vi "VISJS Viewer.vi"(4 "Extra Scripts":string, 5 "FileDependency out":map{path, T1}(c390), 6 "Options":string, 7 "OpenWebBrowser(False)":bool, 8 "error in":errorcluster, 9 "Embedd VISJS Librarya in HTMl File(False)":bool, 10 "HTMLFilePath":path, 11 "LibraryDependency":map{path, T3}(c390)) -> (0 "error out":errorcluster, 3 "HTMLFileContent":string)   [LabVIEW 2020, in "VISJS Viewer.lvlib"]
uses:
  VISJS Viewer.lvlib
  DependencyChecker/LibraryDependentInfo.vi
  <vilib>/Utility/lvfile.llb/FT_FileTypes.ctl
  DependencyChecker/FileDependencyType.ctl
  <vilib>/Utility/miscctls.llb/LVMapReplaceAction.ctl
  <vilib>/Platform/browser.llb/Open URL in Default Browser (path).vi
  <vilib>/Utility/lvfile.llb/NI_FileType.lvlib
  DependencyChecker/DependencyChecker.lvlib
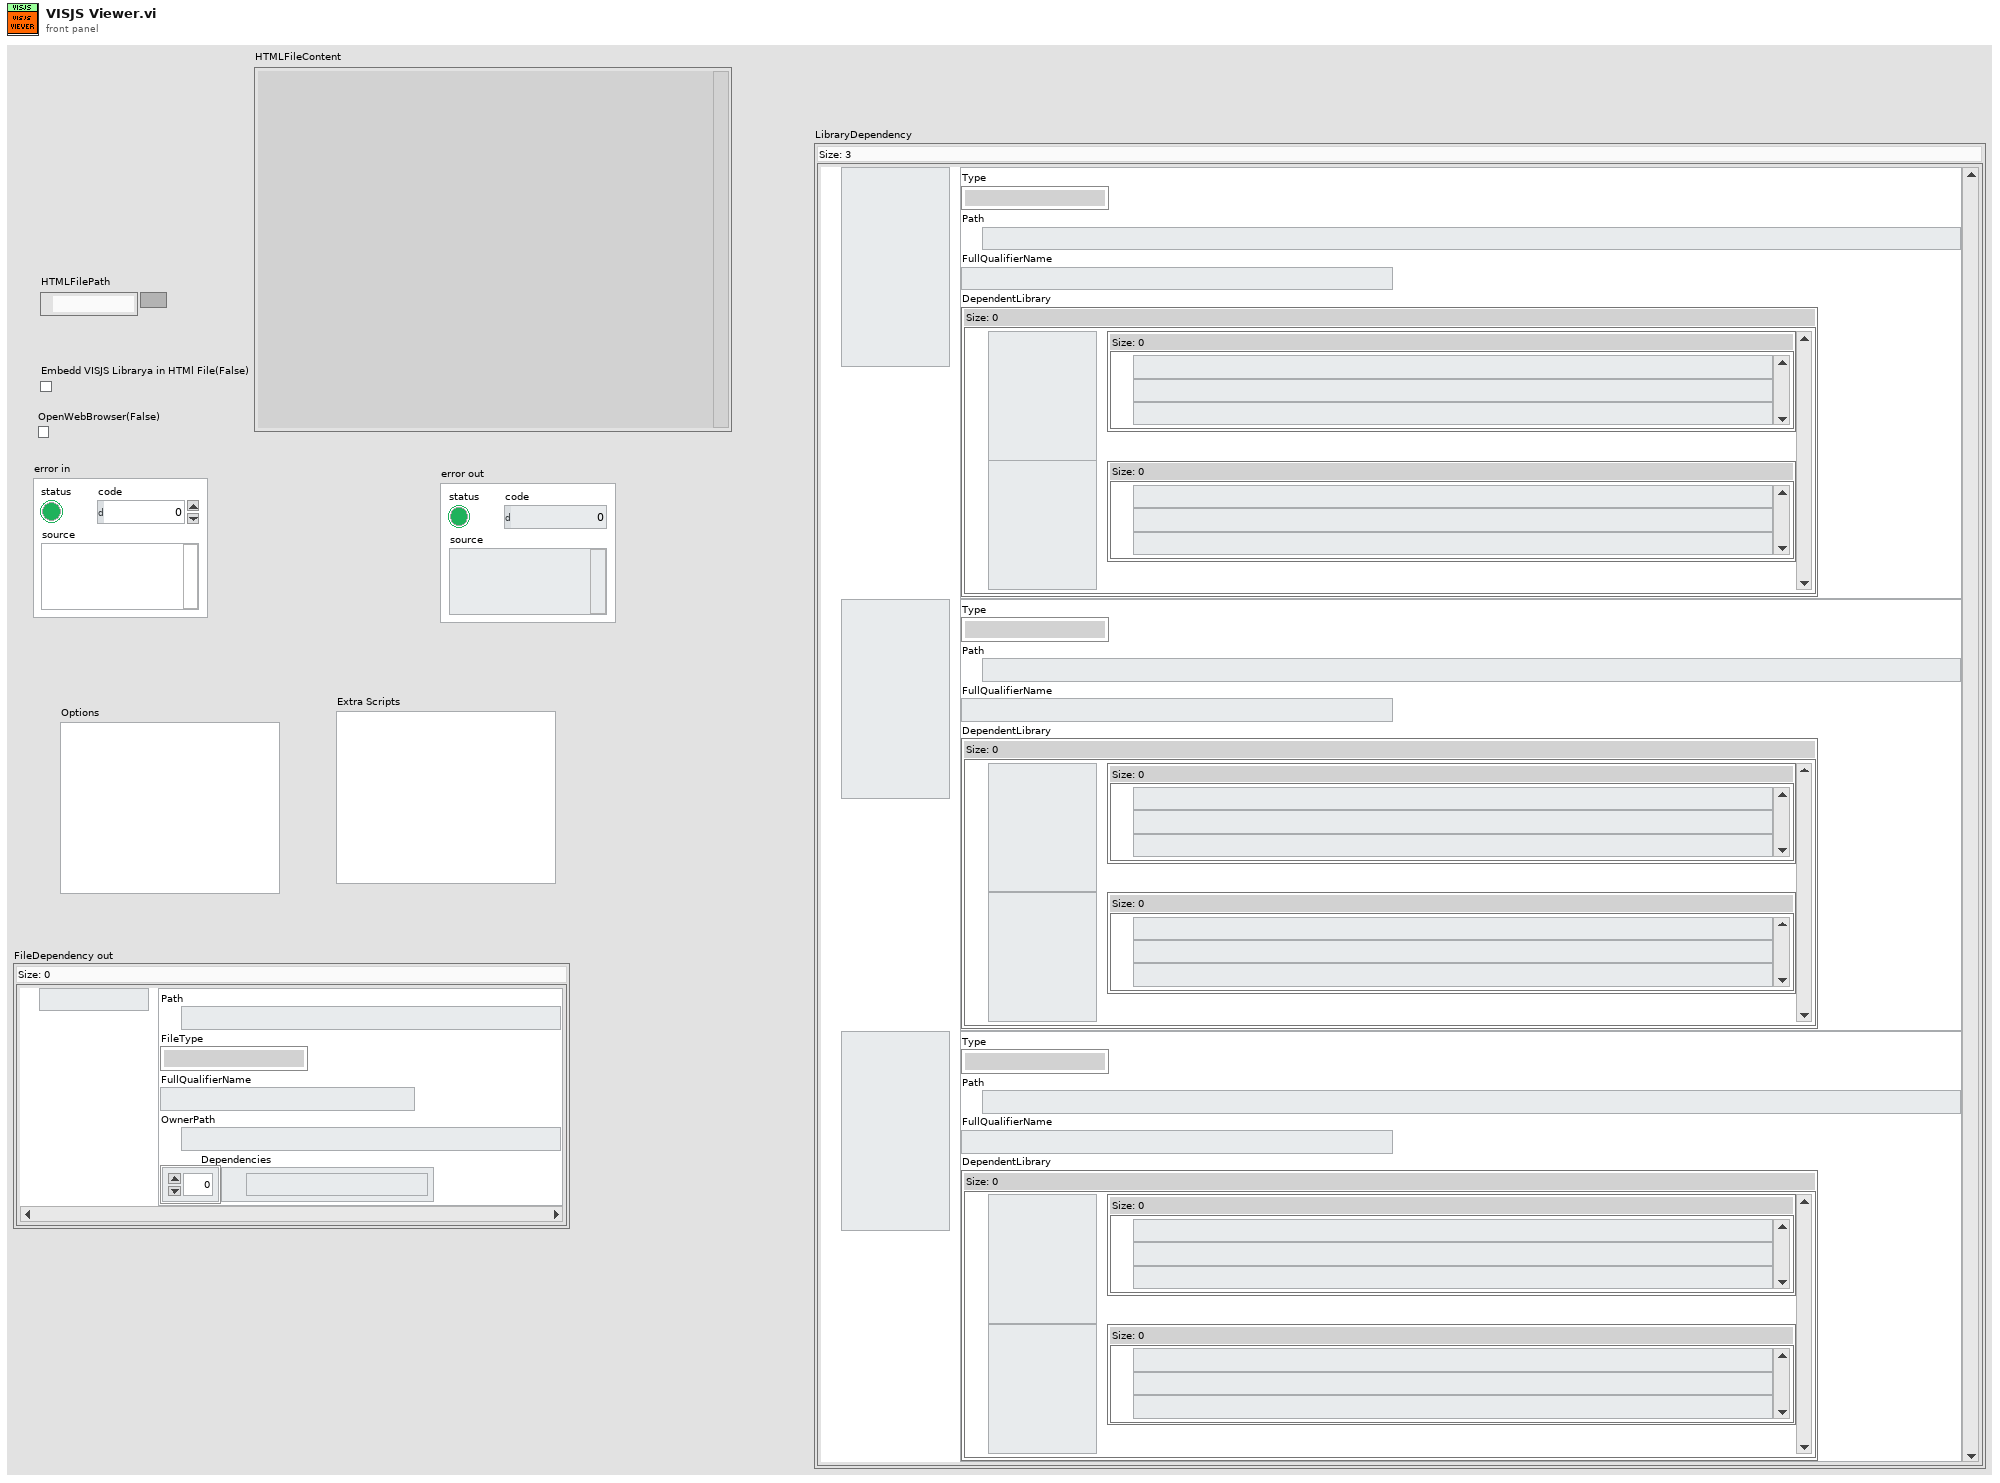
[diagram p1: front panel]
types:
  T1 = typedef "DependencyChecker.lvlib/FileDependencyType.ctl" = cluster{"Path":path, "FileType":T2, "FullQualifierName":string, "OwnerPath":path, "Dependencies":path[]}
  T2 = typedef "NI_FileType.lvlib/FT_FileTypes.ctl" = enum32{"Invalid file/path", "Unknown type", "Instrument", "Control", "Polymorphic VI", "Project", "Library", "LVClass", "XControl", "XNode", "CIN", "Run-time menu", "Palette menu", "LLB", "Shortcut", "Directory", "Class Private Data Control", "Statechart", "MathScript .m file", "Ladder Diagram", "LVLibp"}
  T3 = typedef "DependencyChecker.lvlib/LibraryDependentInfo.vi" = cluster{"Type":T2, "Path":path, "FullQualifierName":string, "DependentLibrary":map{path, set{path}}}
  T4 = typedef "LVMapReplaceAction.ctl" = enum32{"Modify Entry only if found", "Add or Modify Entry", "Delete Entry"}
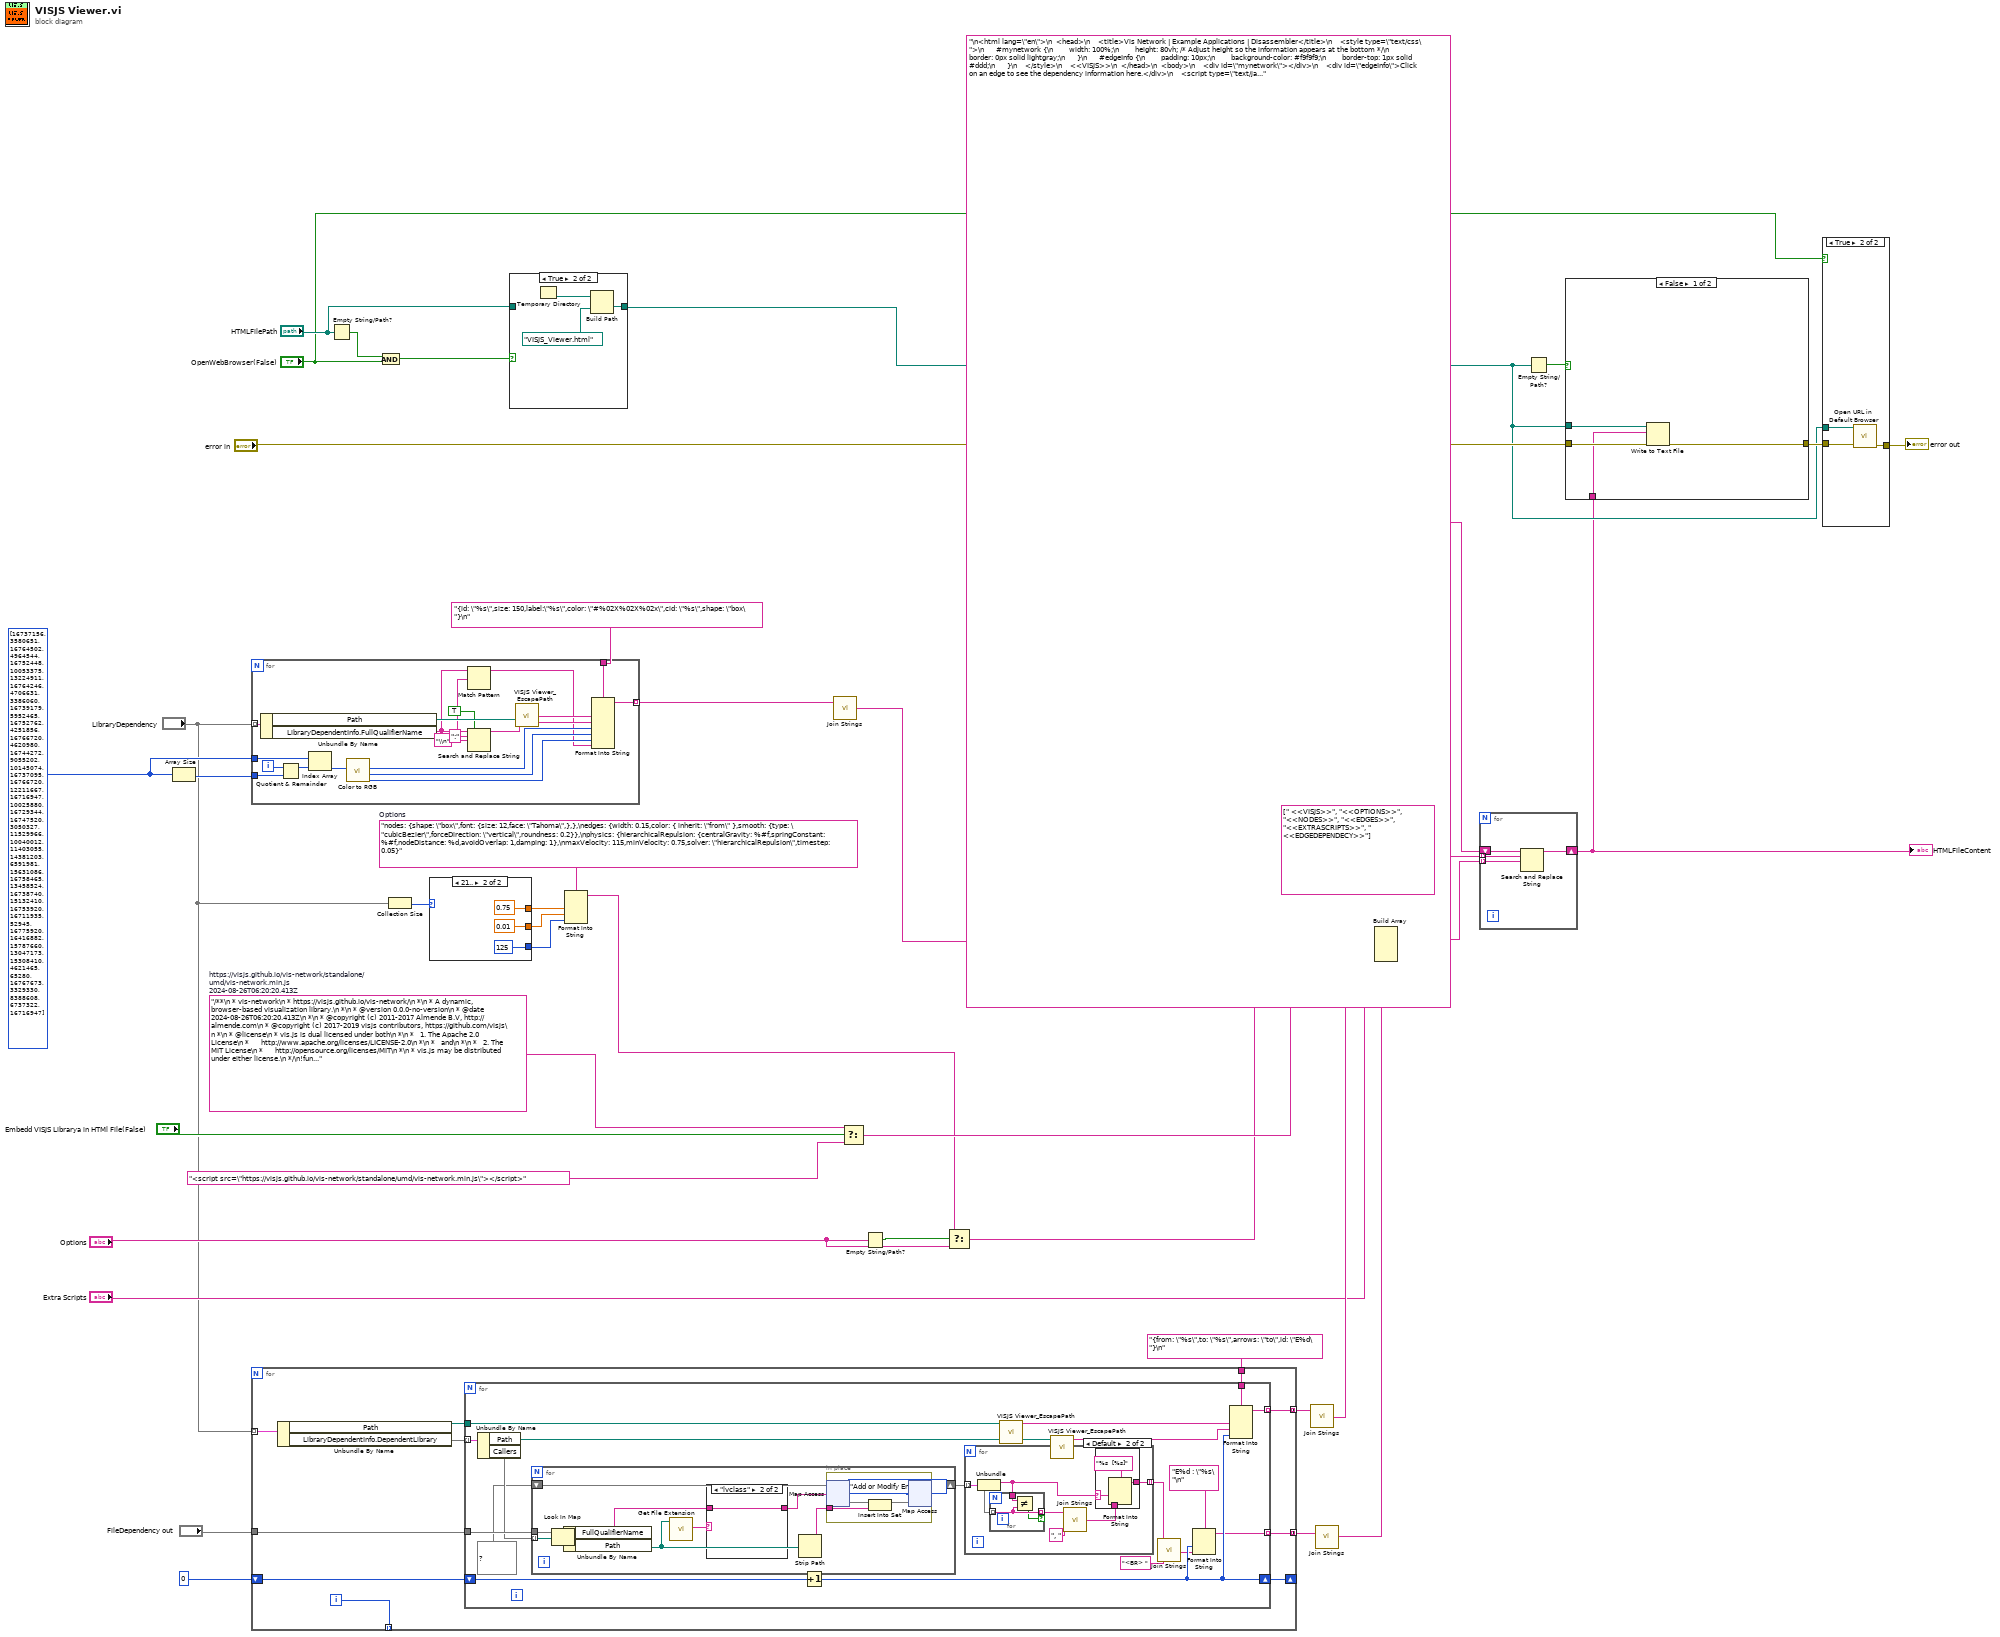
[diagram p0: block diagram]
diagram:
  w28 = u32[] [16737156, 3580651, 16764502, 4964544, 16752448, 10053375, 13224911, 16764246, 4706631, 3386060, 16739179, 5952465, 16752762, 4251856, 16766720, 4620980, 16744272, 9055202, 10145074, 16737095, 16766720, 12211667, 16716947, 10025880, 16729344, 16747520, 3050327, 11529966, 10040012, 11403055, 14381203, 6591981, 15631086, 16758465, 13458524, 16738740, 15132410, 16753920, 16711935, 52945, 16775920, 16416882, 15787660, 13047173, 15308410, 4621465, 65280, 16767673, 3329330, 8388608, 6737322, 16716947] ("Array")
  w9 = "nodes: {shape: \"box\",font: {size: 12,face: \"Tahoma\",},},\nedges: {width: 0.15,color: { inherit: \"from\" },smooth: {type: \"cubicBezier\",forceDirection: \"vertical\",roundness: 0.2}},\nphysics: {hierarchicalRepulsion: {centralGravity: %#f,springConstant: %#f,nodeDistance: %d,avoidOverlap: 1,damping: 1},\nmaxVelocity: 115,minVelocity: 0.75,solver: \"hierarchicalRepulsion\",timestep: 0.05}"  # Options
